vi "PI Query GPIB.vi"(0 "System no.":i32=1 min=1 max=4 step=1, 1 "String to send":string, 2 "Attach Linefeed?":bool=TRUE, 5 "error in":errorcluster) -> (14 "String read":string, 15 "Bytes read":u16, 19 "error out":errorcluster)   [LabVIEW 2013]
doc: "Sub-vi for \"PI Receive String\" for GPIB communication.\n\nValid for C-848, C-880, E-516, F-206, M-8X0 (but must be present in Communication.llb for all other systems, too)"
uses:
  <userlib>/E710_GCS_LabVIEW/Low Level/Communication.llb/Global1.vi
panel:
  out "GPIB configuration":T1={"bus"=0, "address"=4, "mode"=0, "Timeout"=5000}
  # "This vi queries the system via GPIB."
  # "Communication setup indicators (for troubleshooting):"
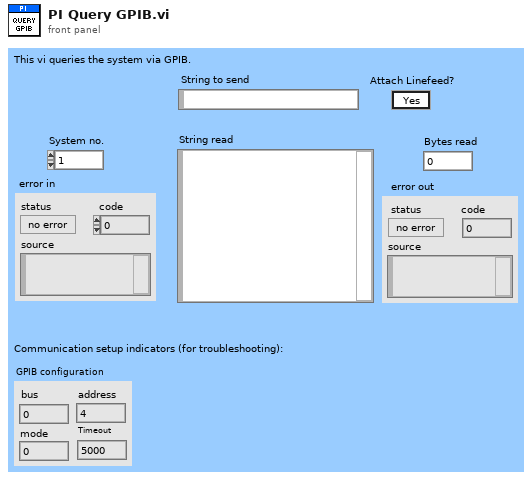
[diagram p1: front panel]
types:
  T1 = cluster{"bus":i16, "address":i16, "mode":i16, "Timeout":u32}
  T2 = cluster{"RS232 Portnumber":u16, "Timeout":u32, "RS232 Baud rate":u32, "Interface":u16, "GPIB Bus":i32, "GPIB Address":i32, "GPIB Mode":i32}[]
  T3 = cluster{"RS232 Portnumber":u16, "Timeout":u32, "RS232 Baud rate":u32, "Interface":u16, "GPIB Bus":i32, "GPIB Address":i32, "GPIB Mode":i32}
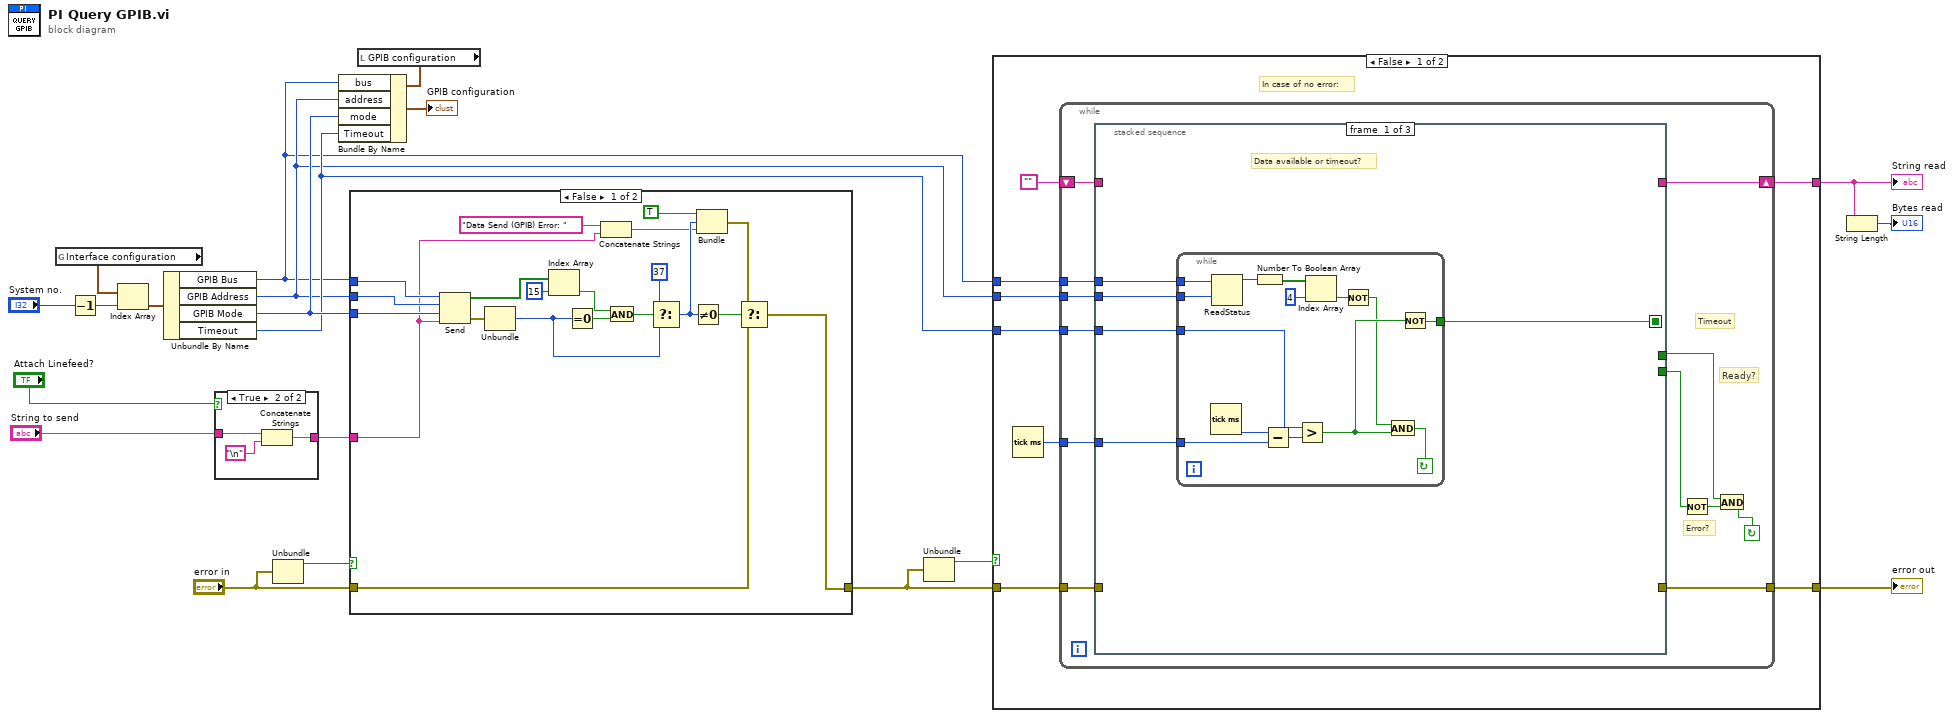
[diagram p0: block diagram]
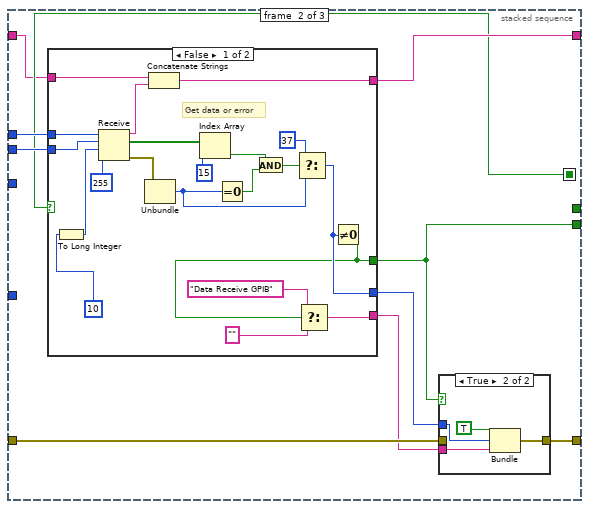
[diagram p2: hidden frame]
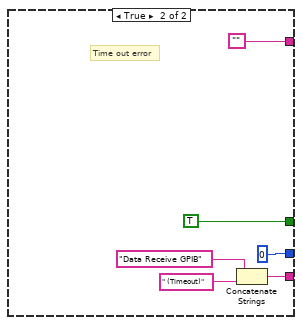
[diagram p4: hidden frame]
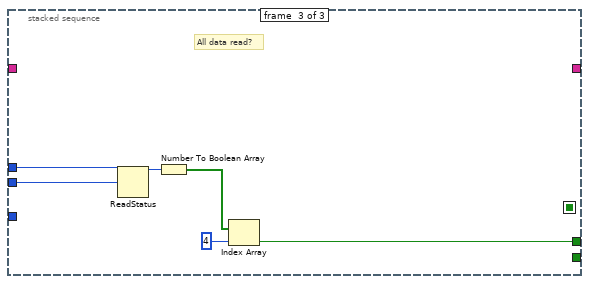
[diagram p5: hidden frame]
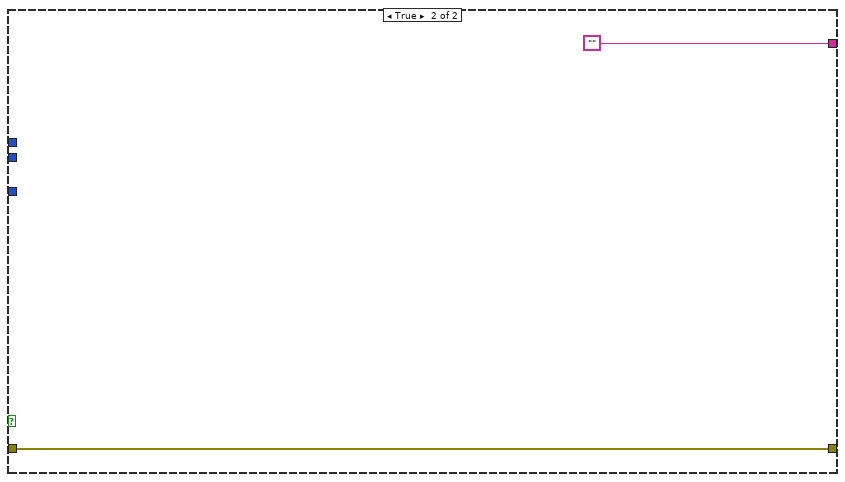
[diagram p6: hidden frame]
diagram:
  n1 = global read "Global1.vi" "Interface configuration"() -> (w17:T2)
  n2 = Decrement(x="System no.") -> (x-1=w15:i32)
  n3 = Index Array(array=w17, index=w15) -> (element=w14:T3)
  n4 = Unbundle By Name(w14) -> ("GPIB Bus"=w3:i32, "GPIB Address"=w4:i32, "GPIB Mode"=w8:i32, "Timeout"=w5:u32)
  n5 = case shown="True" "Attach Linefeed?" {
    tunnel: [w21 w24] -> w9
    tunnel: "String to send" -> [w21 w22]
    frame False {
    }
    frame True {
      n6 = Concatenate Strings(w22, "\n") -> (w24:string)
    }
  }
  n7 = Unbundle("error in") -> ("status"=w19:bool)  [unwired: 2 out]
  n8 = case shown="False" w19 {
    tunnel: "error in" -> [w29 w45]
    tunnel: [w28 w45] -> w7
    tunnel: w3 -> [w30 _]
    tunnel: w4 -> [w31 _]
    tunnel: w9 -> [w25 _]
    tunnel: w8 -> [w32 _]
    frame False {
      n9 = Send(0:w30, 2:w31, 3:w32, 5:w25) -> (6:w39:bool[], 8:w44:errorcluster)  [unwired: 1 in, 1 out]
      n10 = Unbundle(w44) -> ("code"=w37:i32)  [unwired: 2 out]
      n11 = Index Array(array=w39, index=15 ("Index")) -> (element=w38:bool)
      n12 = Equal To 0?(x=w37) -> (x = 0?=w40:bool)
      n13 = Concatenate Strings("Data Send (GPIB) Error: ", w25) -> (w26:string)
      n14 = And(x=w38, y=w40) -> (x .and. y?=w42:bool)
      n15 = Select(t=37, s=w42, f=w37) -> (s? t:f=w35:i32)
      n16 = Not Equal To 0?(x=w35) -> (x != 0?=w34:bool)
      n17 = Bundle(TRUE, "code"=w35, w26) -> (w33:cluster{bool, "code":i32, string})  [unwired: 1 in]
      n18 = Select(t=w33, s=w34, f=w29) -> (s? t:f=w28:errorcluster)
    }
    frame True {
      (unwired) ""
    }
  }
  n19 = local read "GPIB configuration"() -> (w13:T1)
  n20 = Bundle By Name(cluster=w13, "bus"=w3, "address"=w4, "mode"=w8, "Timeout"=w5) -> (→"GPIB configuration":T1)
  n21 = Unbundle(w7) -> ("status"=w6:bool)  [unwired: 2 out]
  n22 = case shown="False" w6 {
    tunnel: w7 -> [w53 w134]
    tunnel: [w52 w134] -> w1
    tunnel: [w46 ""] -> w2
    tunnel: w3 -> [w51 _]
    tunnel: w4 -> [w50 _]
    tunnel: w5 -> [w49 _]
    frame False {
      # "In case of no error:"
      n23 = Tick Count (ms)() -> (millisecond timer value=w48:u32)
      n24 = while {
        tunnel: w53 -> [w65]
        tunnel: [w56] -> w52
        tunnel: w51 -> [w64]
        tunnel: w50 -> [w63]
        tunnel: w49 -> [w62]
        tunnel: w48 -> [w61]
        shift-right: [w59] -> w46
        shift-left: "" -> [w60]
        stop <- w57 continue-if-true
        # "Ready?"
        # "Timeout"
        # "Error?"
        n25 = stacked-sequence {
          seq-local: [w67 _ _] -> [_ w91 _]
          tunnel: w64 -> [w70 w94 w130]
          tunnel: w63 -> [w69 w93 w129]
          tunnel: w62 -> [w68 _ _]
          tunnel: w61 -> [w66 _ _]
          tunnel: [_ w92 _] -> w59
          tunnel: [_ w86 _] -> w56
          tunnel: w65 -> [_ w90 _]
          tunnel: w60 -> [_ w85 _]
          tunnel: [_ w89 _] -> w58
          tunnel: [_ _ w128] -> w55
          frame #0 {
            # "Data available or timeout?"
            n26 = while {
              tunnel: [w77] -> w67
              tunnel: w66 -> [w76]
              tunnel: w70 -> [w75]
              tunnel: w69 -> [w74]
              tunnel: w68 -> [w73]
              stop <- w78 continue-if-true
              n27 = Tick Count (ms)() -> (millisecond timer value=w80:u32)
              n28 = ReadStatus(4:w74, 5:w75) -> (2:w84:i16)  [unwired: 1 in, 2 out]
              n29 = Number To Boolean Array(number=w84) -> (Boolean array=w83:bool[])
              n30 = Subtract(x=w80, y=w76) -> (x-y=w79:u32)
              n31 = Greater?(x=w73, y=w79) -> (0:w72:bool)
              n32 = Index Array(array=w83, index=4) -> (element=w81:bool)
              n33 = Not(x=w81) -> (.not. x?=w71:bool)
              n34 = And(x=w71, y=w72) -> (x .and. y?=w78:bool)
              n35 = Not(x=w72) -> (.not. x?=w77:bool)
            }
          }
          frame #1 {
            n36 = case shown="False" w91 {
              tunnel: [w104 ""] -> w92
              tunnel: w94 -> [w120 _]
              tunnel: w93 -> [w119 _]
              tunnel: [w110 w123] -> w87
              tunnel: [w107 0] -> w88
              tunnel: w85 -> [w106 _]
              tunnel: [w101 TRUE] -> w89
              frame False {
                # "Get data or error"
                n37 = To Long Integer(number=10) -> (32bit integer=w100:i32)
                n38 = Receive(6:255 ("count"), 7:w100, 8:w119, 9:w120) -> (0:w113:errorcluster, 2:w112:bool[], 3:w105:string)  [unwired: 1 in, 1 out]
                n39 = Unbundle(w113) -> ("code"=w111:i32)  [unwired: 2 out]
                n40 = Concatenate Strings(w106, w105) -> (w104:string)
                n41 = Index Array(array=w112, index=15) -> (element=w117:bool)
                n42 = Equal To 0?(x=w111) -> (x = 0?=w118:bool)
                n43 = And(x=w117, y=w118) -> (x .and. y?=w116:bool)
                n44 = Select(t=37, s=w116, f=w111) -> (s? t:f=w107:i32)
                n45 = Not Equal To 0?(x=w107) -> (x != 0?=w101:bool)
                n46 = Select(t="Data Receive GPIB", s=w101, f="") -> (s? t:f=w110:string)
              }
              frame True {
                # "Time out error"
                n47 = Concatenate Strings("Data Receive GPIB", " (Timeout)") -> (w123:string)
              }
            }
            n48 = case shown="True" w89 {
              tunnel: w90 -> [w95 _]
              tunnel: [w95 w99] -> w86
              tunnel: w88 -> [_ w97]
              tunnel: w87 -> [_ w96]
              frame False {
              }
              frame True {
                n49 = Bundle(TRUE, "code"=w97, w96) -> (w99:cluster{bool, "code":i32, string})  [unwired: 1 in]
              }
            }
          }
          frame #2 {
            # "All data read?"
            n50 = ReadStatus(4:w129, 5:w130) -> (2:w131:i16)  [unwired: 1 in, 2 out]
            n51 = Number To Boolean Array(number=w131) -> (Boolean array=w127:bool[])
            n52 = Index Array(array=w127, index=4) -> (element=w128:bool)
          }
        }
        n53 = Not(x=w58) -> (.not. x?=w54:bool)
        n54 = And(x=w55, y=w54) -> (x .and. y?=w57:bool)
      }
    }
    frame True {
    }
  }
  "error out" <- w1
  "String read" <- w2
  n55 = String Length(string=w2) -> (length=→"Bytes read":i32)
